vi "Moving.vi"(10 "Input":variant, 11 "Data in":waveform(dbl)[](array[waveform])) -> (1 "Incorrect movement":bool, 2 "Correct movement":bool, 3 "Centered":bool)   [LabVIEW 2010]
uses:
  <vilib>/Analysis/3filter.llb/Butterworth Filter (DBL).vi
  <vilib>/Analysis/NI_AALBase.lvlib
panel:
  in  "threshold":dbl
  out "Waveform Chart 3":waveform(dbl)(graph)
  in  "high cutoff freq: fh":dbl=50.0
  in  "lowpass cutoff":dbl=200.0
  out "Waveform Chart 2":waveform(dbl)[](graph)
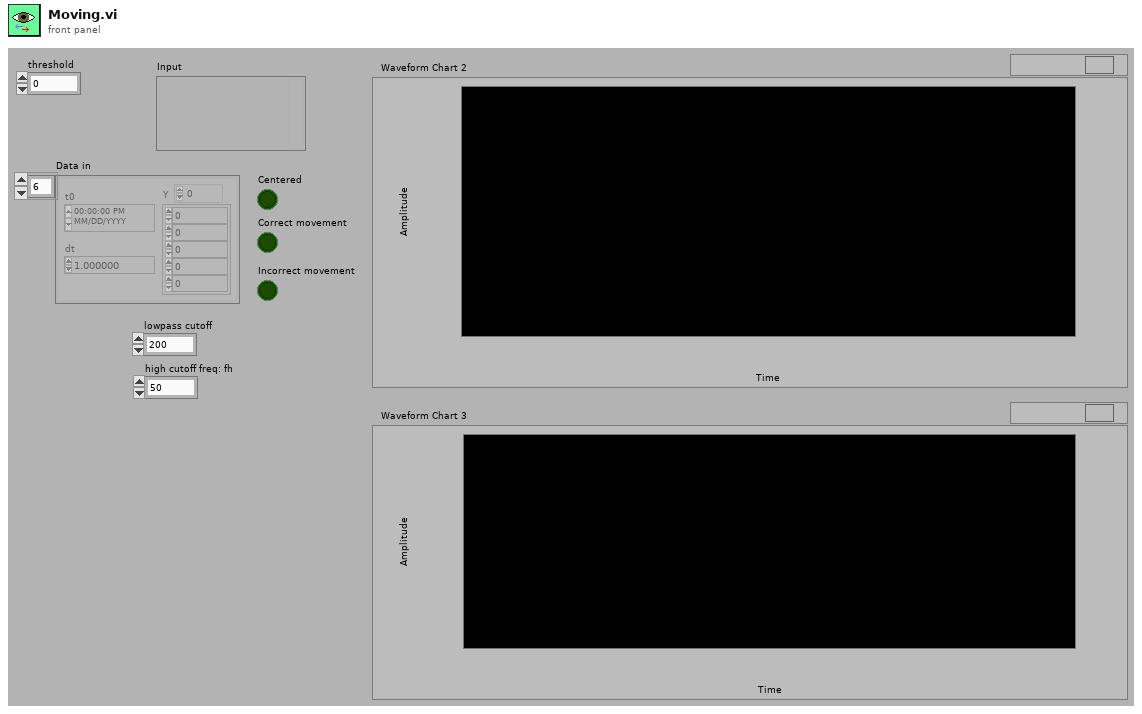
[diagram p1: front panel]
types:
  T1 = enum32{"Lowpass", "Highpass", "Bandpass", "Bandstop"}
  T2 = cluster{"Trial Type":i32, "Joystick Threshold":dbl, "Fixation Radius":dbl}
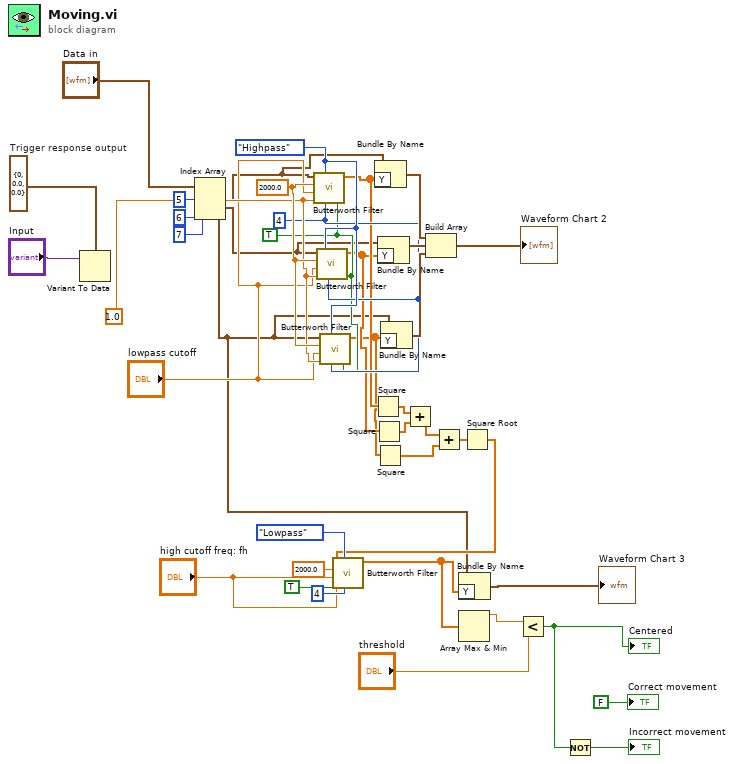
[diagram p0: block diagram]
diagram:
  w30 = 1.0 ("low cutoff freq: fl")
  w29 = 4 ("order")
  w32 = T1."Highpass" ("filter type")
  w28 = TRUE ("init/cont (init:F)")
  w31 = 2000.0 ("sampling freq: fs")
  w39 = T2 {"Trial Type"=0, "Joystick Threshold"=0.0, "Fixation Radius"=0.0}  # Trigger response output
  n1 = Variant To Data(Variant="Input", type=w39) -> ()  [unwired: 1 in, 2 out]
  n2 = Index Array(array="Data in", index #1=5 ("index"), index #2=6 ("index"), index #3=7 ("index")) -> (element #1=w1:waveform(dbl), element #2=w2:waveform(dbl), element #3=w3:waveform(dbl))
  n3 = call-poly <vilib>:"Butterworth Filter.vi"("init/cont (init:F)"=w28, "order"=w29, "filter type"=w32, "low cutoff freq: fl"=w30, "high cutoff freq: fh"="lowpass cutoff", "sampling freq: fs"=w31, "X"=w1) -> ("Filtered X"=w27:dbl[])  [unwired: 2 out]
  n4 = call-poly <vilib>:"Butterworth Filter.vi"("init/cont (init:F)"=w28, "order"=w29, "filter type"=w32, "low cutoff freq: fl"=w30, "high cutoff freq: fh"="lowpass cutoff", "sampling freq: fs"=w31, "X"=w2) -> ("Filtered X"=w26:dbl[])  [unwired: 2 out]
  n5 = call-poly <vilib>:"Butterworth Filter.vi"("init/cont (init:F)"=w28, "order"=w29, "filter type"=w32, "low cutoff freq: fl"=w30, "high cutoff freq: fh"="lowpass cutoff", "sampling freq: fs"=w31, "X"=w3) -> ("Filtered X"=w25:dbl[])  [unwired: 2 out]
  n6 = Square(x=w27) -> (x^2=w24:dbl[])
  n7 = Square(x=w26) -> (x^2=w23:dbl[])
  n8 = Bundle By Name(cluster=w1, "Y"=w27) -> (w35:waveform(dbl))
  n9 = Square(x=w25) -> (x^2=w21:dbl[])
  n10 = Bundle By Name(cluster=w2, "Y"=w26) -> (w34:waveform(dbl))
  n11 = Bundle By Name(cluster=w3, "Y"=w25) -> (w33:waveform(dbl))
  n12 = Add(x=w24, y=w23) -> (x+y=w22:dbl[])
  n13 = Build Array(w35, w34, w33) -> (→"Waveform Chart 2":waveform(dbl)[])
  n14 = Add(x=w22, y=w21) -> (x+y=w20:dbl[])
  n15 = Square Root(x=w20) -> (sqrt(x)=w13:dbl[])
  n16 = call-poly <vilib>:"Butterworth Filter.vi"("init/cont (init:F)"=TRUE, "order"=4, "filter type"=T1."Lowpass", "low cutoff freq: fl"="high cutoff freq: fh", "high cutoff freq: fh"="high cutoff freq: fh", "sampling freq: fs"=2000.0, "X"=w13) -> ("Filtered X"=w9:dbl[])  [unwired: 2 out]
  n17 = Bundle By Name(cluster=w3, "Y"=w9) -> (→"Waveform Chart 3":waveform(dbl))
  n18 = Array Max & Min(array=w9) -> (max value=w8:dbl)  [unwired: 3 out]
  n19 = Less?(x=w8, y="threshold") -> (x < y?=w4:bool)
  "Centered" <- w4
  n20 = Not(x=w4) -> (.not. x?=→"Incorrect movement":bool)
  "Correct movement" <- FALSE ("Correct movement")
